vi "waveformgraphexample.vi"() -> ()   [LabVIEW 2015]
panel:
  out "x0 =0":dbl[](graph)
  out "Cluster waveform graph":cluster{dbl, dbl, dbl[]}(graph)
  in  "stop":bool
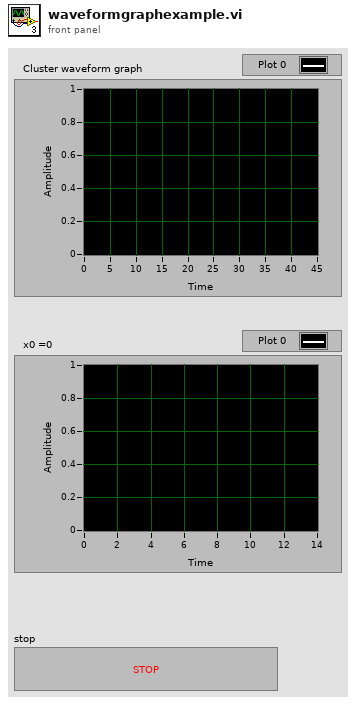
[diagram p1: front panel]
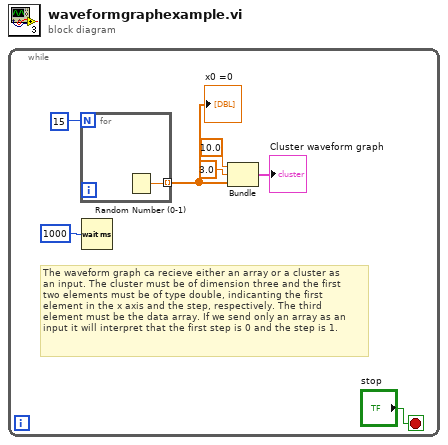
[diagram p0: block diagram]
diagram:
  n1 = while {
    stop <- "stop" stop-if-true
    # "The waveform graph ca recieve either an array or a cluster as\nan input. The cluster must be of dimension three and the first\ntwo elements must be of type double, indicanting the first \nelement in the x axis and the step, respectively. The third\nelement must be the data array. If we send only an array as an\ninput it will interpret that the first step is 0 and the step is 1."
    n2 = for {
      N: 15 -> [_]
      tunnel: [w8] -> w5 mode=indexing
      n3 = Random Number (0-1)() -> (number: 0 to 1=w8:dbl)
    }
    "x0 =0" <- w5
    n4 = Wait (ms)(milliseconds to wait=u32 1000) -> ()  [unwired: 1 out]
    n5 = Bundle(10.0, 3.0, w5) -> (→"Cluster waveform graph":cluster{dbl, dbl, dbl[]})  [unwired: 1 in]
  }
